vi "sslSimulationProtocolDecodeRobotsFeedback.vi"(8 "error in (no error)":errorcluster, 10 "Key":i32=2, 11 "robotsFeedbackArray":u8[](array[numeric])) -> (0 "error out":errorcluster, 3 "RobotsFeedback":refnum<class "RobotFeedback.lvclass">[](array[class]))   [LabVIEW 2023, in "Communication.lvclass"]
uses:
  Communication.lvclass
  RobotFeedback/RobotFeedback.lvclass
panel:
  out "Communication out":refnum<class "Communication.lvclass">
  in  "Communication in":refnum<class "Communication.lvclass">
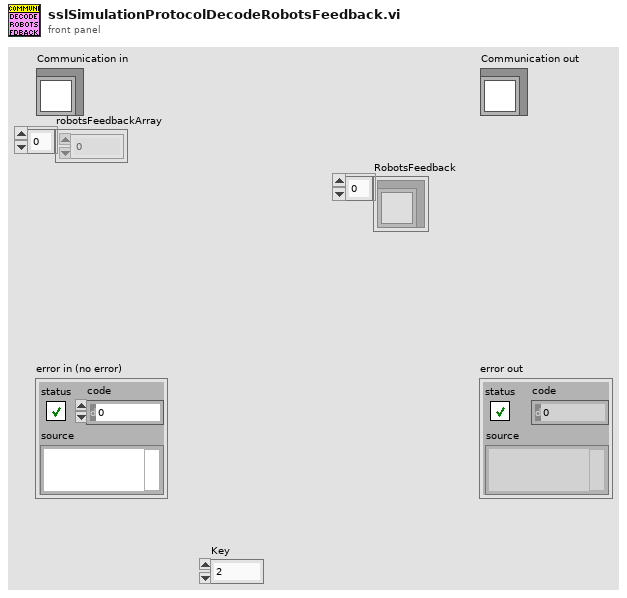
[diagram p1: front panel]
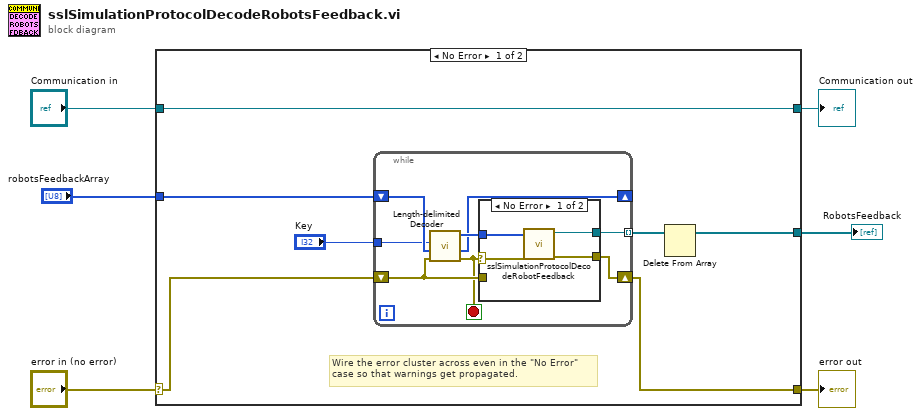
[diagram p0: block diagram]
diagram:
  n1 = case shown="No Error" "error in (no error)" {
    selector: "error in (no error)" -> [w10 w28]
    tunnel: [w9 w28] -> w5
    tunnel: [w13 w27] -> w3
    tunnel: "Communication in" -> [w13 w27]
    tunnel: "robotsFeedbackArray" -> [w11 _]
    tunnel: [w7 _] -> w1
    frame No Error {
      # "Wire the error cluster across even in the \"No Error\"\ncase so that warnings get propagated."
      n2 = while {
        shift-right: [w19] -> _
        shift-left: w11 -> [w16]
        shift-right: [w21] -> w9
        shift-left: w10 -> [w18]
        tunnel: "Key" -> [w15]
        tunnel: [w14] -> w8 mode=indexing
        stop <- w17 stop-if-true
        n3 = call "Length-delimited Decoder.vi"("error in (no error)"=w18, "Array"=w16, "Key"=w15) -> ("error out"=w17:errorcluster, "array w/ subset deleted"=w19:u8[], "Length-delimited"=w20:u8[])  [unwired: 5 in, 1 out]
        n4 = case shown="No Error" w17 {
          selector: w17 -> [w24 _]
          tunnel: [w23 w26] -> w21
          tunnel: w20 -> [w25 _]
          tunnel: w18 -> [_ w26]
          tunnel: [w22 _] -> w14
          frame No Error {
            n5 = call "sslSimulationProtocolDecodeRobotFeedback.vi"("error in (no error)"=w24, "robotFeedbackArray"=w25) -> ("error out"=w23:errorcluster, "RobotFeedback.lvclass"=w22:refnum<class "RobotFeedback.lvclass">)  [unwired: 8 in]
          }
          frame Error {
          }
        }
      }
      n6 = Delete From Array(array=w8) -> (array with subset deleted=w7:refnum<class "RobotFeedback.lvclass">[])  [unwired: 2 in, 1 out]
    }
    frame Error {
    }
  }
  "error out" <- w5
  "Communication out" <- w3
  "RobotsFeedback" <- w1
